vi "XML.vi"() -> ()   [LabVIEW 2023]
uses:
  <vilib>/xml/NI_XML.lvlib
  <resource>/objmgr/DOMUserDefRef.rc
panel:
  out "output array":string[](array[string])
  in  "XPath expression":string
  in  "error in (no error)":errorcluster
  out "XML":string
  out "Parse Errors":string
  in  "Schedule Filename":string
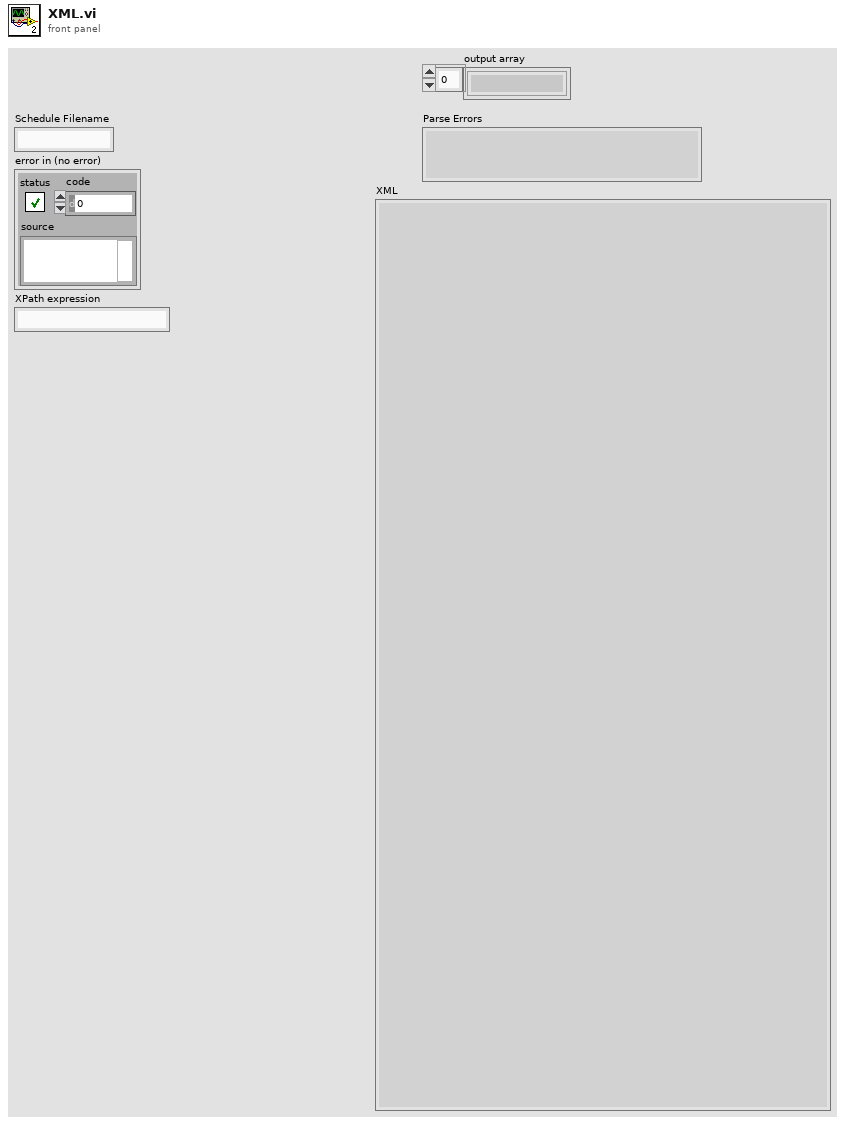
[diagram p1: front panel]
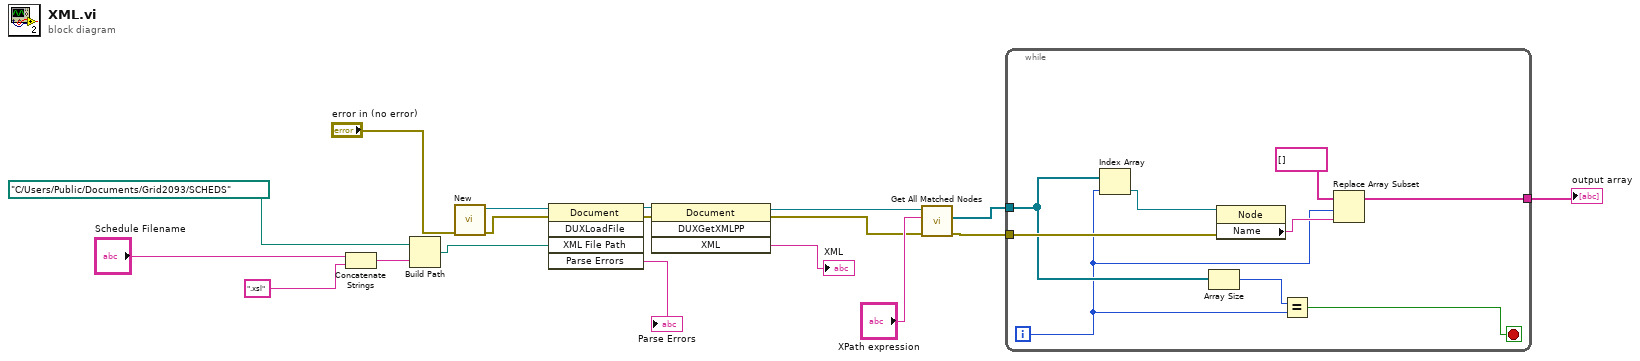
[diagram p0: block diagram]
diagram:
  n1 = Concatenate Strings("Schedule Filename", ".xsl" ("string")) -> (w11:string)
  n2 = Build Path(base path=path "C:/Users/Public/Documents/Grid2093/SCHEDS", name or relative path=w11) -> (appended path=w8:path)
  n3 = call <vilib>:"New.vi"("error in (no error)"="error in (no error)") -> ("error out"=w17:errorcluster, "DOM document out"=w18:refnum<k20>)  [unwired: 7 in]
  n4 = invoke class="Document" method="DUXLoadFile"(reference=w18, error in=w17, "XML File Path"=w8) -> (reference out=w16:refnum<k20>, error out=w15:errorcluster, "Parse Errors"=→"Parse Errors":string)  [unwired: 2 in, 2 out]
  n5 = invoke class="Document" method="DUXGetXMLPP"(reference=w16, error in=w15) -> (reference out=w4:refnum<k20>, error out=w3:errorcluster, "XML"=→"XML":string)  [unwired: 2 in, 1 out]
  n6 = call <vilib>:"Get All Matched Nodes.vi"("error in (no error)"=w3, "XPath expression"="XPath expression", "node in"=w4) -> ("error out"=w5:errorcluster, "node result array"=w2:refnum<k20>[])  [unwired: 6 in, 1 out]
  n7 = while {
    tunnel: w5 -> [w27]
    tunnel: w2 -> [w25]
    tunnel: [w19] -> w1
    i -> [w21]
    stop <- w23 stop-if-true
    n8 = Index Array(array=w25, index=w21) -> (element=w26:refnum<k20>)
    n9 = Array Size(array=w25) -> (size(s)=w24:i32)
    n10 = property class="Node"(reference=w26, error in=w27) -> ("Name"=w22:string)  [unwired: 2 out]
    n11 = Equal?(x=w24, y=w21) -> (x = y?=w23:bool)
    n12 = Replace Array Subset(array=string[] [], new element=w22, index=w21) -> (w19:string[])
  }
  "output array" <- w1
